vi "ALTS-2015 Read Write Cluster for Last Saved Results.vi"(4 "advisory dialog? (display:T)":bool, 5 "Prompt":string, 6 "Option":enum16{"Read", "Write"}(ring), 7 "pattern(*.set)":string="*.set", 8 "error in (no error)":errorcluster, 10 "Cluster In":T1, 11 "File path":path) -> (0 "error out":errorcluster, 2 "Cluster Out":T1, 3 "File path out":path)   [LabVIEW 2013]
doc: "This VI reads (or writes) the cluster from (to) the specified file.\n\nCopyright © 2005, Soliton Technologies.\nAll rights reserved."
uses:
  Controls/ALTS-2015 Read Write Cluster Last Saved Results Data cluster.ctl
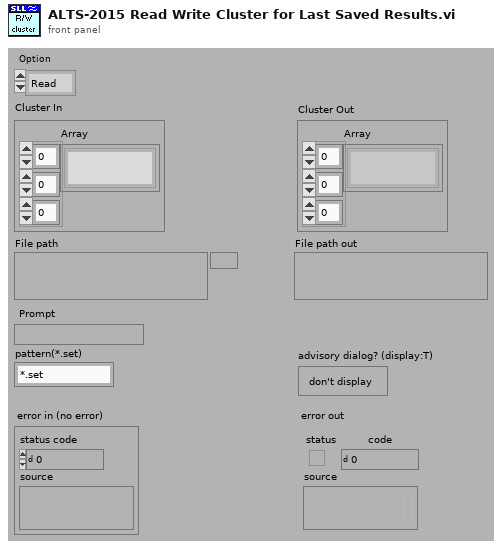
[diagram p1: front panel]
types:
  T1 = typedef "ALTS-2015 Read Write Cluster Last Saved Results Data cluster.ctl" = cluster{"Array":string[][][]}
  T2 = enum16{"open", "open or create", "create or replace", "create"}
  T3 = enum16{"open", "open or create", "create or replace", "create", "open (read only)"}
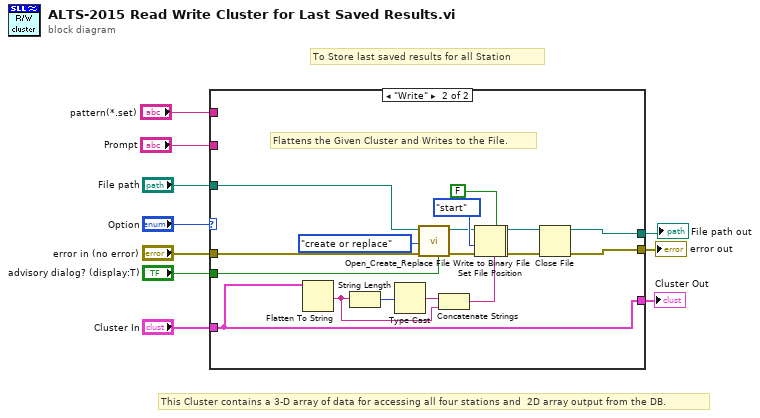
[diagram p0: block diagram]
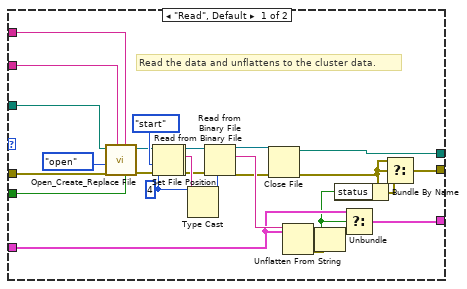
[diagram p2: hidden frame]
diagram:
  # "This Cluster contains a 3-D array of data for accessing all four stations and  2D array output from the DB."
  # "To Store last saved results for all Station"
  n1 = case shown="\"Write\"" "Option" {
    tunnel: "File path" -> [w26 w48]
    tunnel: [w15 w50] -> w9
    tunnel: "error in (no error)" -> [w25 w47]
    tunnel: "Cluster In" -> [w20 w49]
    tunnel: [w18 w49] -> w1
    tunnel: "advisory dialog? (display:T)" -> [w24 w44]
    tunnel: "Prompt" -> [w23 _]
    tunnel: "pattern(*.set)" -> [w22 _]
    tunnel: [w21 w43] -> w2
    frame "Read", Default {
      w36 = 4 ("count")
      # "Read the data and unflattens to the cluster data."
      n2 = call <vilib>:"Open_Create_Replace File.vi"("advisory dialog? (display:T)"=w24, "pattern"=w22, "prompt"=w23, "error in (no error)"=w25, "function (open:0)"=T2."open", "file path"=w26) -> ("error out"=w32:errorcluster, "refnum"=w30:refnum<file>)  [unwired: 2 in, 2 out]
      n3 = Set File Position(refnum=w30, from (0:start)=enum16{"start", "end", "current"}."start" ("pos mode (0:2)"), error in=w32) -> (refnum out=w13:refnum<file>, error out=w12:errorcluster)  [unwired: 1 in]
      n4 = Read from Binary File(8:w12, 10:w36, 11:w13) -> (0:w34:errorcluster, 2:w35:string, 3:w33:refnum<file>)  [unwired: 3 in, 1 out]
      n5 = Type Cast(type=w36, x=w35) -> (*(type *) &x=w37:i32)
      n6 = Read from Binary File(8:w34, 10:w37, 11:w33) -> (0:w27:errorcluster, 2:w38:string, 3:w28:refnum<file>)  [unwired: 3 in, 1 out]
      n7 = Close File(refnum=w28, error in=w27) -> (path=w21:path, error out=w16:errorcluster)
      n8 = Unflatten From String(type=w20, binary string=w38) -> (value=w19:T1, error out=w11:errorcluster)  [unwired: 3 in, 1 out]
      n9 = Unbundle(w11) -> ("status"=w17:bool)  [unwired: 2 out]
      n10 = Bundle By Name(cluster=w16, "status"=w17) -> (w14:errorcluster)
      n11 = Select(t=w20, s=w17, f=w19) -> (s? t:f=w18:T1)
      n12 = Select(t=w16, s=w16, f=w14) -> (s? t:f=w15:errorcluster)
    }
    frame "Write" {
      # "Flattens the Given Cluster and Writes to the File."
      n13 = Flatten To String(anything=w49) -> (data string=w55:string)  [unwired: 3 in, 2 out]
      n14 = String Length(string=w55) -> (length=w57:i32)
      n15 = Type Cast(x=w57) -> (*(type *) &x=w56:string)  [unwired: 1 in]
      n16 = call <vilib>:"Open_Create_Replace File.vi"("advisory dialog? (display:T)"=w44, "error in (no error)"=w47, "function (open:0)"=T3."create or replace", "file path"=w48) -> ("error out"=w45:errorcluster, "refnum"=w46:refnum<file>)  [unwired: 4 in, 2 out]
      n17 = Concatenate Strings(w56, w55) -> (w54:string)
      n18 = Set File Position(refnum=w46, from (0:start)=enum16{"start", "end", "current"}."start" ("pos mode (0:2)"), error in=w45) -> (refnum out=w41:refnum<file>, error out=w40:errorcluster)  [unwired: 1 in]
      n19 = Write to Binary File(file (use dialog)=w41, data=w54, error in=w40, 5:FALSE ("prepend array or string size? (T)")) -> (refnum out=w52:refnum<file>, error out=w51:errorcluster)  [unwired: 2 in, 1 out]
      n20 = Close File(refnum=w52, error in=w51) -> (path=w43:path, error out=w50:errorcluster)
    }
  }
  "error out" <- w9
  "File path out" <- w2
  "Cluster Out" <- w1
